vi "Apex Valve Program.vi"() -> ()   [LabVIEW 2009]
panel:
  out "CASE":T1(ring)
  in  "Tab Control 2":enum32{"Display", "XY Graph", "Setup"}(tab)
  out "ON/OFF":bool
  in  "Start Warmup":bool
  in  "ON Time (s)":dbl=5.0
  in  "OFF Time (s)":dbl=15.0
  in  "Cycle Limit":i32=100
  in  "Test Details":T2
  out "Time Remaining (s)":dbl=-5.1021575927734375e-05 format="%.1f"
  out "Cycle Count":i32=1
  out "# of Rows Saved":i32
  out "Waveform Chart":waveform(dbl)(graph)
  out "File Path Output":path=path "X:/DISP/LabVIEW-Shared/Blake Otting/Apex Valve Program/Data/ApexValve-4-15-2010-{7-PM}.xls"
  in  "FAIL Button":bool
  in  "PASS Button":bool
  in  "Start Test":bool
  in  "Max Elapsed Build Time (ms)":u32=5000
  in  "Build Interval (ms)":u32=1
  in  "High Trigger SP (VDC)":dbl=3.0
  in  "Use Trigger SP?":bool=TRUE
  out "Array Size":i32=2993
  out "XY Graph":cluster{u32[], dbl[]}(graph)
  in  "Tab Control":T3(tab)
  out "Analog Error":errorcluster
  out "Analog Task":refnum<k21>="SC1Mod3"
  in  "Analog Module Config":T4={"DAQ #"=1, "Module #"=3, "Samples"=1, "Mode"=12522, "Rate (Hz)"=500.0, "Min VDC"=-10.0, "Max VDC"=32.0, "Module Type"=enum."SCXI"} {"Rate (Hz)" format="%0.2f"; "Mode" items=["Finite Samples"=10178, "Continuous Samples"=10123, "Hardware Timed Single Point"=12522]}
  in  "Digital Output Module Configure":T5={"Module Type"=enum."SCXI", "DAQ #"=1, "Module #"=2}
  out "Digital Task":refnum<k21>="SC1Mod2"
  out "Digital Error":errorcluster
  out "Event Loop":i32
  out "DAQ Loop":i32=1452
  out "File Save Error":errorcluster caption="Error Output"
  out "Main Loop":i32=11302
  in  "STOP PROGRAM":bool
  # "Created by Blake Otting\nApril 15th 2010"
  # "APEX VALVE PROGRAM"
  # "Warm Up Settings"
  # "Test Settings"
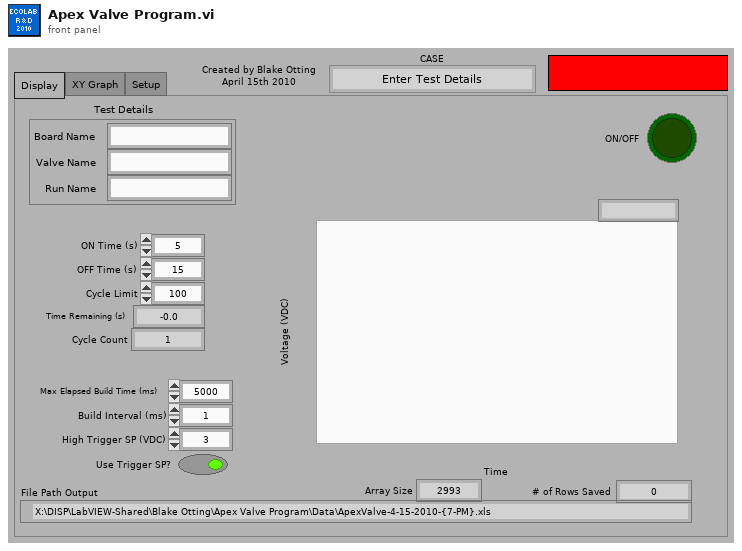
[diagram p1: front panel]
types:
  T1 = enum16{"Enter Test Details", "Warm-Up Cycles", "Test Mode", "Evaluate & Save"}
  T2 = cluster{"Board Name":string, "Valve Name":string, "Run Name":string}
  T3 = enum32{"Analog Input", "Digital Output", "Program"}
  T4 = cluster{"DAQ #":i32, "Module #":i32, "Samples":i32, "Mode":i32, "Rate (Hz)":dbl, "Min VDC":dbl, "Max VDC":dbl, "Module Type":enum16{"CDAQ", "SCXI"}}
  T5 = cluster{"Module Type":enum16{"CDAQ", "SCXI"}, "DAQ #":i32, "Module #":i32}
  T6 = cluster{"Row Limit":i32, "Default File Name":string, "New File Daily?":bool, "Manual Save Interval?":bool}
  T7 = cluster{"Elapsed (ms)":u32, "Voltage (VDC)":dbl}[]
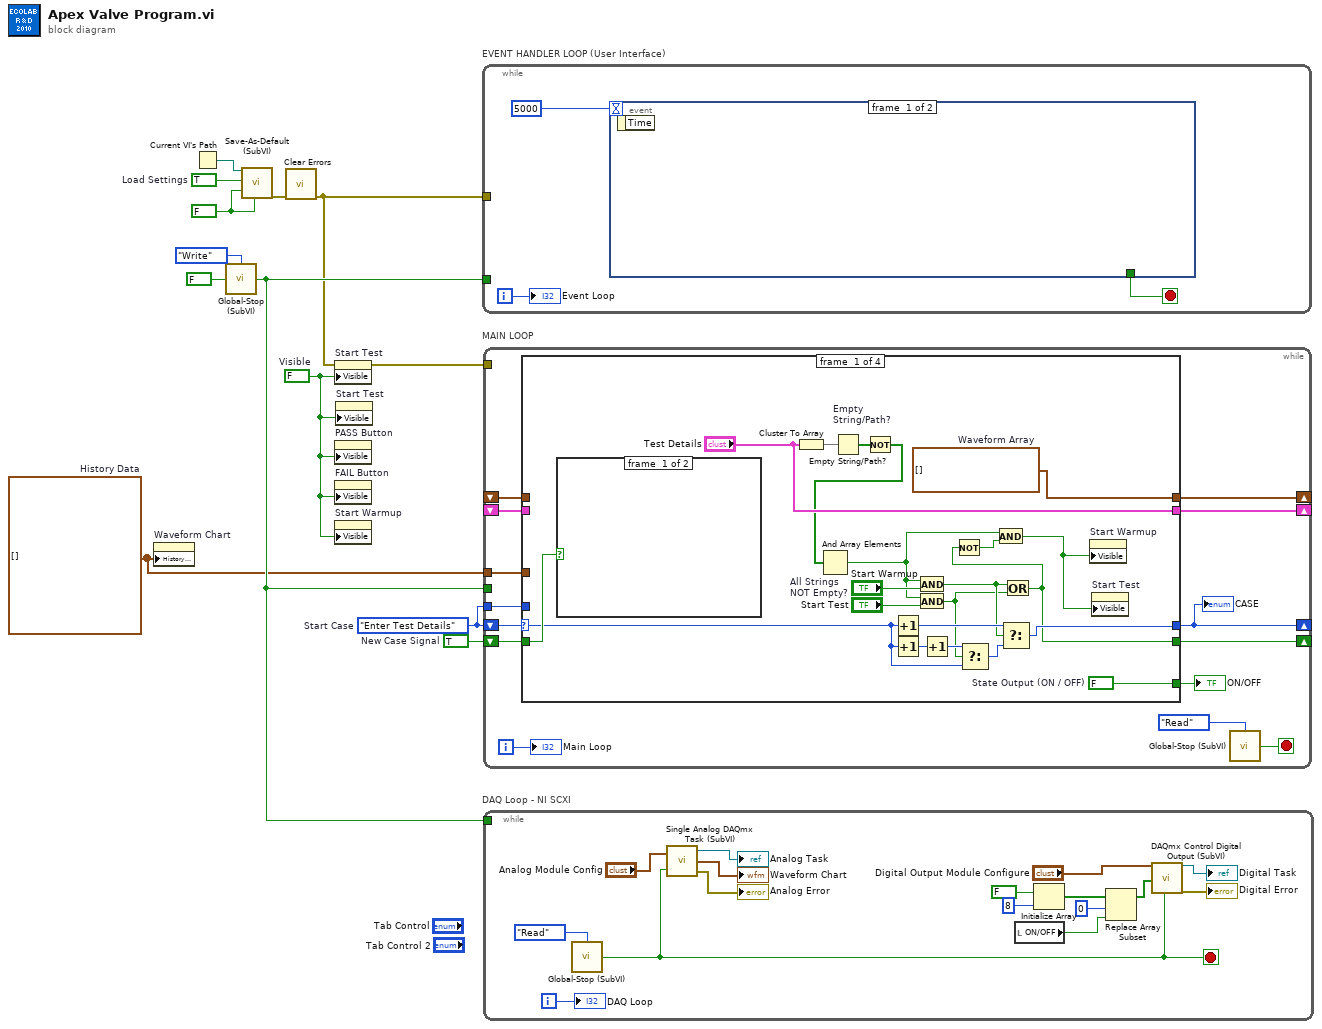
[diagram p0: block diagram]
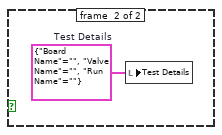
[diagram p2: hidden frame]
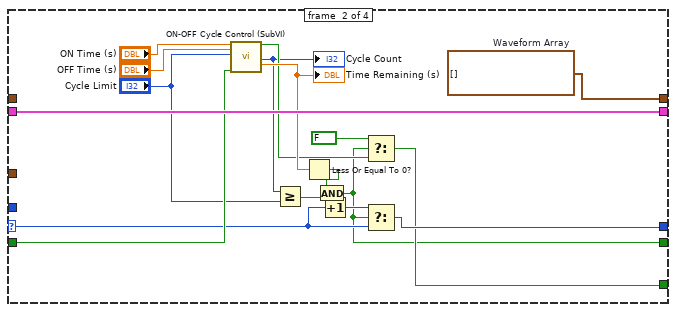
[diagram p3: hidden frame]
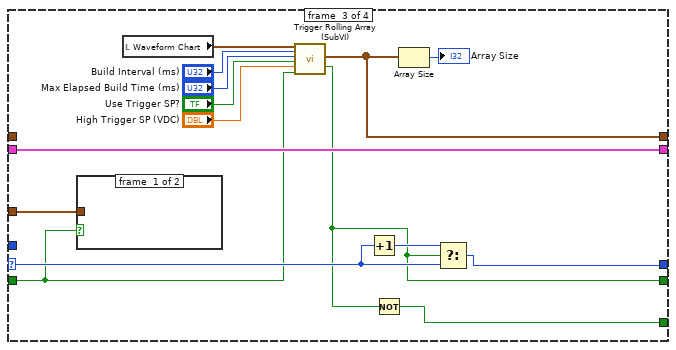
[diagram p4: hidden frame]
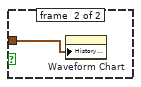
[diagram p5: hidden frame]
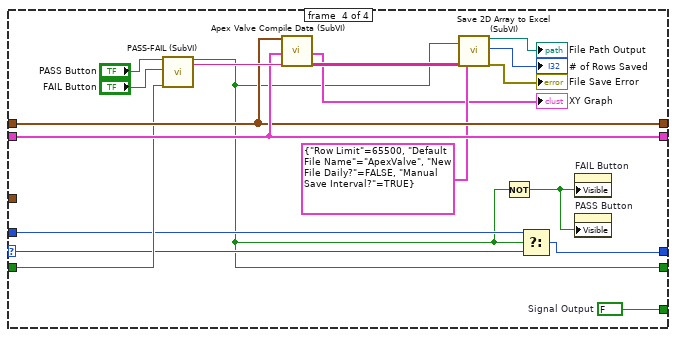
[diagram p6: hidden frame]
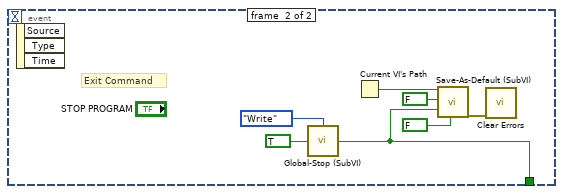
[diagram p7: hidden frame]
diagram:
  w3 = waveform(dbl)[] []  # History Data
  w1 = FALSE  # Visible
  w7 = TRUE  # New Case Signal
  w2 = T1."Enter Test Details"  # Start Case
  w9 = FALSE ("Save Settings")
  w10 = TRUE  # Load Settings
  n1 = property on="Waveform Chart" class="WFChart (strict)"("History Data"=w3) -> ()  [unwired: 2 in, 2 out]
  n2 = Current VI's Path() -> (path=w11:path)
  n3 = call "Global-Stop (SubVI).vi"("Mode (Read)"=enum16{"Read", "Write"}."Write", "IN"=FALSE) -> ("OUT"=w8:bool)  [unwired: 2 out]
  n4 = call "Save-As-Default (SubVI).vi"("Current VI's Path"=w11, "Load Settings"=w10, "Save Settings"=w9, "Save and Exit"=w9) -> ("Save as Default Error"=w5:errorcluster)  [unwired: 15 in]
  n5 = call <vilib>:"Clear Errors.vi"("error in (no error)"=w5) -> ("error out"=w4:errorcluster)  [unwired: 6 out]
  n6 = property on="Start Test" class="Bool (strict)"(error in=w4, "Visible"=w1) -> (error out=w6:errorcluster)  [unwired: 1 in, 1 out]
  n7 = property on="PASS Button" class="Bool (strict)"("Visible"=w1) -> ()  [unwired: 2 in, 2 out]
  n8 = property on="FAIL Button" class="Bool (strict)"("Visible"=w1) -> ()  [unwired: 2 in, 2 out]
  n9 = property on="Start Warmup" class="Bool (strict)"("Visible"=w1) -> ()  [unwired: 2 in, 2 out]
  n10 = property on="Start Test" class="Bool (strict)"("Visible"=w1) -> ()  [unwired: 2 in, 2 out]
  n11 = while "EVENT HANDLER LOOP (User Interface)" {
    tunnel: w8 -> [_]
    tunnel: w4 -> [_]
    i -> [w14]
    stop <- w16 stop-if-true
    n12 = event shown="[1] \"STOP PROGRAM\": Mouse Down;  Panel Close" {
      selector: _ -> [_ _]
      dyn-events: _ -> [_ _]
      timeout: 5000 ("Event Loop Wait (ms)") -> [_ _]
      tunnel: [_ w18] -> w16
      event #0 {
        n13 = event-data() -> ()  [unwired: 2 out]
      }
      event #1 {
        # "Exit Command"
        n14 = event-data() -> ()  [unwired: 4 out]
        n15 = call "Global-Stop (SubVI).vi"("Mode (Read)"=enum16{"Read", "Write"}."Write", "IN"=TRUE) -> ("OUT"=w18:bool)  [unwired: 2 out]
        n16 = Current VI's Path() -> (path=w20:path)
        n17 = call "Save-As-Default (SubVI).vi"("Current VI's Path"=w20, "Load Settings"=FALSE, "Save Settings"=w18, "Save and Exit"=FALSE ("Save Settings")) -> ("Save as Default Error"=w17:errorcluster)  [unwired: 15 in]
        n18 = call <vilib>:"Clear Errors.vi"("error in (no error)"=w17) -> ()  [unwired: 7 out]
      }
    }
    "Event Loop" <- w14
  }
  n19 = while "MAIN LOOP" {
    tunnel: w8 -> [_]
    shift-right: [w28] -> _
    shift-left: w2 -> [w34]
    shift-right: [w27] -> _
    shift-left: w7 -> [w33]
    shift-right: [w32] -> _
    shift-left: _ -> [w31]
    shift-right: [w30] -> _
    shift-left: _ -> [w29]
    tunnel: w6 -> [_]
    tunnel: w3 -> [w25]
    tunnel: w2 -> [w24]
    i -> [w35]
    stop <- w36 stop-if-true
    n20 = case shown="\"Test Mode\"" w34 {
      selector: w34 -> [w48 w69 w88 w97]
      tunnel: w33 -> [w54 w72 w85 w102]
      tunnel: [w58 w76 w81 w106] -> w32
      tunnel: w31 -> [_ _ _ w106]
      tunnel: ["Test Details" w75 w91 w107] -> w30
      tunnel: w29 -> [_ w75 w91 w107]
      tunnel: [w47 w70 w87 w95] -> w28
      tunnel: [w40 w60 w82 w94] -> w27
      tunnel: [w53 w65 w83 w105] -> w26
      tunnel: w25 -> [_ _ w84 _]
      tunnel: w24 -> [_ _ _ w96]
      frame #0 {
        w53 = FALSE  # State Output (ON / OFF)
        w58 = T7 []  # Waveform Array
        n21 = case shown="True" w54 {
          frame #0 {
          }
          frame #1 {
            w59 = T2 {"Board Name"="", "Valve Name"="", "Run Name"=""}  # Test Details
            n22 = local write "Test Details"(w59) -> ()
          }
        }
        n23 = Cluster To Array(cluster="Test Details") -> (array=w56:string[])
        n24 = Empty String/Path? "Empty \nString/Path?"(string/path=w56) -> (empty?=w55:bool[])
        n25 = Not(x=w55) -> (.not. x?=w44:bool[])
        n26 = And Array Elements "All Strings\nNOT Empty?"(Boolean array=w44) -> (logical AND=w41:bool)
        n27 = Increment(x=w48) -> (x+1=w52:T1)
        n28 = Increment(x=w48) -> (x+1=w50:T1)
        n29 = And(x=w41, y="Start Warmup") -> (x .and. y?=w43:bool)
        n30 = And(x=w41, y="Start Test") -> (x .and. y?=w42:bool)
        n31 = Increment(x=w50) -> (x+1=w49:T1)
        n32 = Select(t=w49, s=w42, f=w48) -> (s? t:f=w51:T1)
        n33 = Select(t=w52, s=w43, f=w51) -> (s? t:f=w47:T1)
        n34 = Or(x=w43, y=w42) -> (x .or. y?=w40:bool)
        n35 = Not(x=w40) -> (.not. x?=w39:bool)
        n36 = And(x=w41, y=w39) -> (x .and. y?=w38:bool)
        n37 = property on="Start Warmup" class="Bool (strict)"("Visible"=w38) -> ()  [unwired: 2 in, 2 out]
        n38 = property on="Start Test" class="Bool (strict)"("Visible"=w38) -> ()  [unwired: 2 in, 2 out]
      }
      frame #1 {
        w76 = T7 []  # Waveform Array
        n39 = call "ON-OFF Cycle Control (SubVI).vi"("ON Time (s)"="ON Time (s)", "OFF Time (s)"="OFF Time (s)", "Cycle Limit"="Cycle Limit", "Reset Cycle Count"=w72) -> ("State Output (ON / OFF)"=w66:bool, "Cycle Count"=w64:i32, "Time Remaining (s)"=w68:dbl)  [unwired: 11 in, 2 out]
        "Cycle Count" <- w64
        "Time Remaining (s)" <- w68
        n40 = Greater Or Equal?(x=w64, y="Cycle Limit") -> (x >= y?=w61:bool)
        n41 = Less Or Equal To 0?(x=w68) -> (x <= 0?=w62:bool)
        n42 = And(x=w62, y=w61) -> (x .and. y?=w60:bool)
        n43 = Increment(x=w69) -> (x+1=w71:T1)
        n44 = Select(t=FALSE, s=w60, f=w66) -> (s? t:f=w65:bool)
        n45 = Select(t=w71, s=w60, f=w69) -> (s? t:f=w70:T1)
      }
      frame #2 {
        n46 = case shown="True" w85 {
          tunnel: w84 -> [_ w92]
          frame #0 {
          }
          frame #1 {
            n47 = property on="Waveform Chart" class="WFChart (strict)"("History Data"=w92) -> ()  [unwired: 2 in, 2 out]
          }
        }
        n48 = local read "Waveform Chart"() -> (w86:waveform(dbl))
        n49 = call "Trigger Rolling Array (SubVI).vi"("Waveform Input"=w86, "Build Interval (ms)"="Build Interval (ms)", "Max Elapsed Build Time (ms)"="Max Elapsed Build Time (ms)", "Use Trigger SP?"="Use Trigger SP?", "High Trigger SP (VDC)"="High Trigger SP (VDC)", "Clear Trigger SP Latch"=w85) -> ("Waveform Array"=w81:T7, "Build Array Complete?"=w82:bool)  [unwired: 12 in]
        n50 = Increment(x=w88) -> (x+1=w89:T1)
        n51 = Not(x=w82) -> (.not. x?=w83:bool)
        n52 = Array Size(array=w81) -> (size(s)=→"Array Size":i32)
        n53 = Select(t=w89, s=w82, f=w88) -> (s? t:f=w87:T1)
      }
      frame #3 {
        w105 = FALSE  # Signal Output
        n54 = call "PASS-FAIL (SubVI).vi"("PASS Button"="PASS Button", "FAIL Button"="FAIL Button", "Clear PASS/FAIL Selection"=w102) -> ("PASS/FAIL Latch"=w94:bool, "PASS/FAIL String"=w108:string)  [unwired: 12 in, 3 out]
        n55 = call "Apex Valve Compile Data (SubVI).vi"("Waveform Array Input"=w106, "Test Details"=w107, "PASS/FAIL"=w108) -> ("XY Graph"=→"XY Graph":cluster{u32[], dbl[]}, "2D Data Array"=w104:string[][])  [unwired: 15 in]
        n56 = call "Save 2D Array to Excel (SubVI).vi"("Save (Enable/Signal)"=w94, "Data Array (Table)"=w104, "File Configuration"=T6 {"Row Limit"=65500, "Default File Name"="ApexValve", "New File Daily?"=FALSE, "Manual Save Interval?"=TRUE}) -> ("File Path Output"=→"File Path Output":path, "# of Rows Saved"=→"# of Rows Saved":i32, "Error Output"=→"File Save Error":errorcluster)  [unwired: 13 in, 1 out]
        n57 = Not(x=w94) -> (.not. x?=w93:bool)
        n58 = Select(t=w96, s=w94, f=w97) -> (s? t:f=w95:T1)
        n59 = property on="FAIL Button" class="Bool (strict)"("Visible"=w93) -> ()  [unwired: 2 in, 2 out]
        n60 = property on="PASS Button" class="Bool (strict)"("Visible"=w93) -> ()  [unwired: 2 in, 2 out]
      }
    }
    "ON/OFF" <- w26
    "CASE" <- w28
    n61 = call "Global-Stop (SubVI).vi"("Mode (Read)"=enum16{"Read", "Write"}."Read") -> ("OUT"=w36:bool)  [unwired: 1 in, 2 out]
    "Main Loop" <- w35
  }
  n62 = while "DAQ Loop - NI SCXI" {
    tunnel: w8 -> [_]
    i -> [w125]
    stop <- w120 stop-if-true
    n63 = call "Global-Stop (SubVI).vi"("Mode (Read)"=enum16{"Read", "Write"}."Read") -> ("OUT"=w120:bool)  [unwired: 1 in, 2 out]
    n64 = call "Single Analog DAQmx Task (SubVI).vi"("Module Configure"="Analog Module Config", "E-STOP Input"=w120) -> ("Task OUT"=→"Analog Task":refnum<k21>, "Waveform Output"=→"Waveform Chart":waveform(dbl), "Error OUT"=→"Analog Error":errorcluster)
    n65 = local read "ON/OFF"() -> (w116:bool)
    n66 = Initialize Array(FALSE ("Pump Relay State"), 8 ("dimension size")) -> (w115:bool[])
    n67 = Replace Array Subset(array=w115, new element=w116, index=0) -> (w112:bool[])
    n68 = call "DAQmx Control Digital Output (SubVI).vi"("Digital Output Module Configure"="Digital Output Module Configure", "Relay Control"=w112, "E-STOP Input"=w120) -> ("Task OUT"=→"Digital Task":refnum<k21>, "Error OUT"=→"Digital Error":errorcluster)  [unwired: 15 in]
    "DAQ Loop" <- w125
  }
